vi "SpecAn Marker Parameters Set.vi"(0 "VISA In":refnum<visa-resource-name>, 5 "Error In":errorcluster, 6 "Readout":i32(ring) items=["Auto", "Frequency", "Period", "Time", "Inverse Time"], 8 "Marker Type":i32(ring) items=["Normal", "Delta", "Fixed", "Off"], 10 "Active Marker":i32(ring)=1 items=["Marker1"=1, "Marker2"=2, "Marker3"=3, "Marker4"=4, "Marker5"=5, "Marker6"=6, "Marker7"=7, "Marker8"=8, "Marker9"=9, "Marker10"=10, "Marker11"=11, "Marker12"=12]) -> (14 "VISA Out":refnum<visa-resource-name>, 19 "Error Out":errorcluster)   [LabVIEW 2015]
uses:
  Controls/FGV Action SpecAn Model.ctl
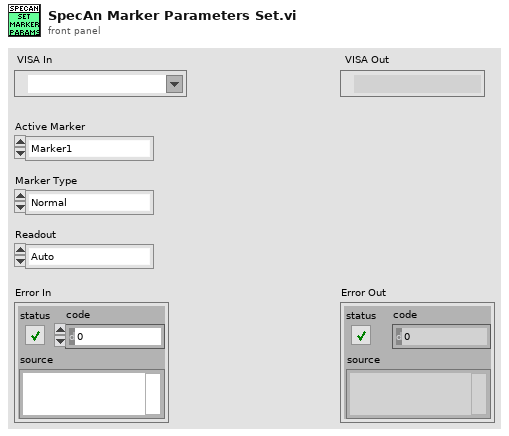
[diagram p1: front panel]
types:
  T1 = typedef "FGV Action SpecAn Model.ctl" = enum16{"Get", "Set"}
  T2 = typedef "SpecAn Model.ctl" = enum16{"E4440", "N9030"}
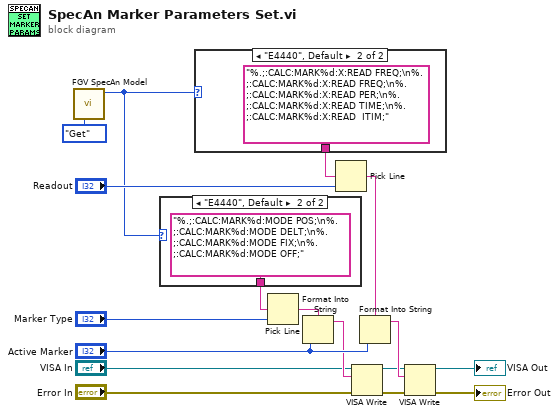
[diagram p0: block diagram]
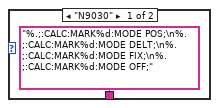
[diagram p2: hidden frame]
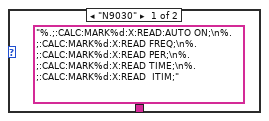
[diagram p3: hidden frame]
diagram:
  n1 = call "FGV SpecAn Model.vi"("Action"=FGV_Action_SpecAn_Model."Get") -> ("SA Model"=w1:T2)  [unwired: 6 in, 1 out]
  n2 = case shown="\"E4440\", Default" w1 {
    tunnel: ["%.;:CALC:MARK%d:MODE POS;\n%.;:CALC:MARK%d:MODE DELT;\n%.;:CALC:MARK%d:MODE FIX;\n%.;:CALC:MARK%d:MODE OFF;" ("Marker Type") "%.;:CALC:MARK%d:MODE POS;\n%.;:CALC:MARK%d:MODE DELT;\n%.;:CALC:MARK%d:MODE FIX;\n%.;:CALC:MARK%d:MODE OFF;" ("Marker Type")] -> w10
    frame "N9030" {
    }
    frame "E4440", Default {
    }
  }
  n3 = case shown="\"E4440\", Default" w1 {
    tunnel: ["%.;:CALC:MARK%d:X:READ:AUTO ON;\n%.;:CALC:MARK%d:X:READ FREQ;\n%.;:CALC:MARK%d:X:READ PER;\n%.;:CALC:MARK%d:X:READ TIME;\n%.;:CALC:MARK%d:X:READ  ITIM;" ("Marker Readout") "%.;:CALC:MARK%d:X:READ FREQ;\n%.;:CALC:MARK%d:X:READ FREQ;\n%.;:CALC:MARK%d:X:READ PER;\n%.;:CALC:MARK%d:X:READ TIME;\n%.;:CALC:MARK%d:X:READ  ITIM;" ("Marker Readout")] -> w14
    frame "N9030" {
    }
    frame "E4440", Default {
    }
  }
  n4 = Pick Line(multi-line string=w10, line index="Marker Type") -> (output string=w15:string)  [unwired: 1 in]
  n5 = Format Into String(format string=w15, "Active Marker") -> (resulting string=w8:string)  [unwired: 2 in, 1 out]
  n6 = Pick Line(multi-line string=w14, line index="Readout") -> (output string=w12:string)  [unwired: 1 in]
  n7 = VISA Write(VISA resource name="VISA In", write buffer=w8, error in (no error)="Error In") -> (VISA resource name out=w4:refnum<visa-resource-name>, error out=w3:errorcluster)  [unwired: 1 out]
  n8 = Format Into String(format string=w12, "Active Marker") -> (resulting string=w7:string)  [unwired: 2 in, 1 out]
  n9 = VISA Write(VISA resource name=w4, write buffer=w7, error in (no error)=w3) -> (VISA resource name out=→"VISA Out":refnum<visa-resource-name>, error out=→"Error Out":errorcluster)  [unwired: 1 out]
